vi "test_GetItemInfosFromProjectFile_SplitProjectTargetsSolution.vi"() -> (3 "Pass?":bool)   [LabVIEW 2019, in "Tests.SolutionBuilder.lvlib"]
uses:
  Tests.SolutionBuilder.lvlib
  SolutionBuilder/SolutionBuilder.lvclass
  SolutionBuilder/ProjectItem/ProjectItem.lvclass
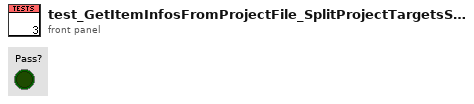
[diagram p1: front panel]
types:
  T1 = typedef "SolutionBuilder.lvlib/SolutionBuilder.lvclass/ProjectItemMap.ctl" = map{path, refnum<class "ProjectItem.lvclass">[]}
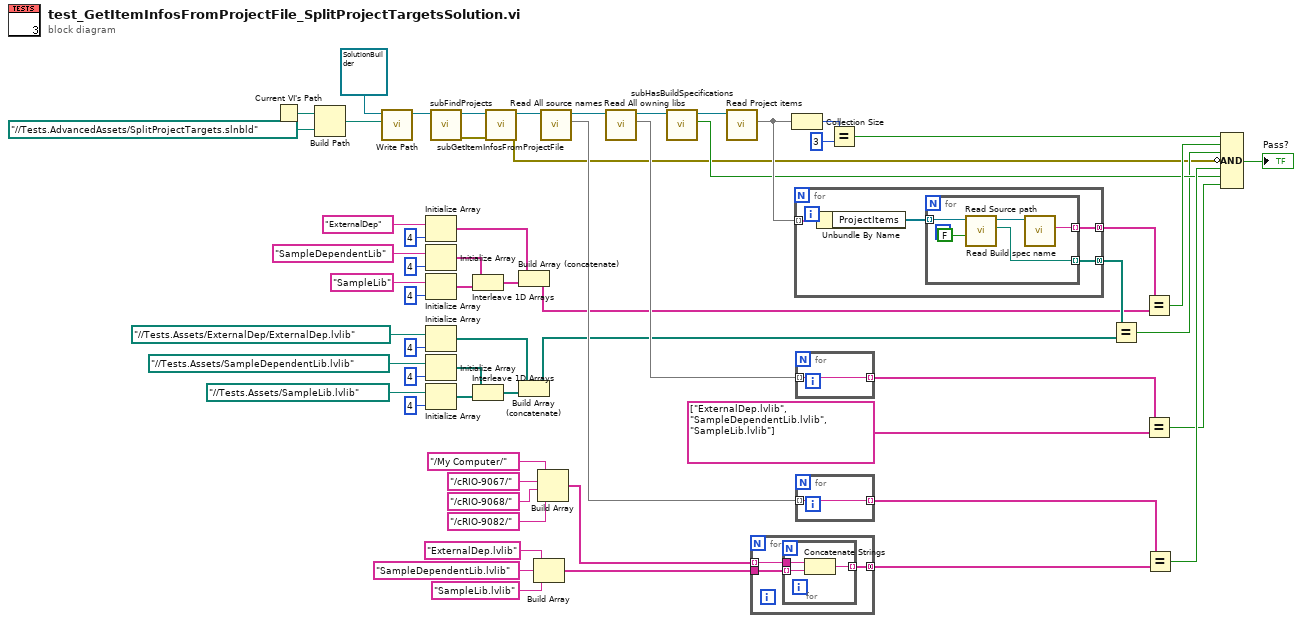
[diagram p0: block diagram]
diagram:
  n1 = Current VI's Path() -> (path=w58:path)
  n2 = Build Path(base path=w58, name or relative path=path "../../Tests.AdvancedAssets/SplitProjectTargets.slnbld" ("Path")) -> (appended path=w56:path)
  n3 = call "Write Path.vi"("Path"=w56, "SolutionBuilder in"=refnum<class "SolutionBuilder.lvclass"> refnum) -> ("SolutionBuilder out"=w60:refnum<class "SolutionBuilder.lvclass">)  [unwired: 9 in]
  n4 = Initialize Array("ExternalDep" ("Build spec name"), 4 ("dimension size")) -> (w24:string[])
  n5 = Initialize Array("SampleDependentLib" ("Build spec name"), 4 ("dimension size")) -> (w27:string[])
  n6 = Initialize Array("SampleLib" ("Build spec name"), 4 ("dimension size")) -> (w26:string[])
  n7 = Initialize Array(path "../../Tests.Assets/ExternalDep/ExternalDep.lvlib" ("Source path"), 4 ("dimension size")) -> (w22:path[])
  n8 = Initialize Array(path "../../Tests.Assets/SampleDependentLib.lvlib" ("Source path"), 4 ("dimension size")) -> (w19:path[])
  n9 = Initialize Array(path "../../Tests.Assets/SampleLib.lvlib" ("Source path"), 4 ("dimension size")) -> (w20:path[])
  n10 = call "subFindProjects.vi"("SolutionBuilder in"=w60) -> ("error out"=w35:errorcluster, "SolutionBuilder out"=w59:refnum<class "SolutionBuilder.lvclass">)  [unwired: 9 in]
  n11 = Interleave 1D Arrays(w27, w26) -> (w25:string[])
  n12 = Interleave 1D Arrays(w19, w20) -> (w21:path[])
  n13 = call "subGetItemInfosFromProjectFile.vi"("error in (no error)"=w35, "SolutionBuilder in"=w59) -> ("error out"=w34:errorcluster, "SolutionBuilder out"=w53:refnum<class "SolutionBuilder.lvclass">)  [unwired: 8 in]
  n14 = Build Array (concatenate)(w24, w25) -> (w23:string[])
  n15 = Build Array (concatenate)(w22, w21) -> (w12:path[])
  n16 = Build Array("ExternalDep.lvlib" ("Build spec name"), "SampleDependentLib.lvlib" ("Build spec name"), "SampleLib.lvlib" ("Build spec name")) -> (w3:string[])
  n17 = Build Array("/My Computer/" ("Build spec name"), "/cRIO-9067/" ("Build spec name"), "/cRIO-9068/" ("Build spec name"), "/cRIO-9082/" ("Build spec name")) -> (w4:string[])
  n18 = call "Read All source names.vi"("SolutionBuilder in"=w53) -> ("All source names"=w49:set{string}, "SolutionBuilder out"=w41:refnum<class "SolutionBuilder.lvclass">)  [unwired: 9 in]
  n19 = call "Read All owning libs.vi"("SolutionBuilder in"=w41) -> ("All owning libs"=w39:set{string}, "SolutionBuilder out"=w40:refnum<class "SolutionBuilder.lvclass">)  [unwired: 9 in]
  n20 = call "subHasBuildSpecifications.vi"("SolutionBuilder in"=w40) -> ("Has specs?"=w46:bool, "SolutionBuilder out"=w47:refnum<class "SolutionBuilder.lvclass">)  [unwired: 8 in, 1 out]
  n21 = call "Read Project items.vi"("SolutionBuilder in"=w47) -> ("Project items"=w52:T1)  [unwired: 9 in, 1 out]
  n22 = for {
    tunnel: w4 -> [w64] mode=indexing
    tunnel: w3 -> [w63]
    tunnel: [w62] -> w2 mode=concatenating
    n23 = for {
      tunnel: w64 -> [w67]
      tunnel: w63 -> [w66] mode=indexing
      tunnel: [w65] -> w62 mode=indexing
      n24 = Concatenate Strings(w67, w66) -> (w65:string)
    }
  }
  n25 = Collection Size(1:w52) -> (0:w55:i32)
  n26 = for {
    tunnel: w52 -> [w71] mode=indexing
    tunnel: [w70] -> w45 mode=concatenating
    tunnel: [w68] -> w43 mode=concatenating
    n27 = Unbundle By Name(w71) -> ("ProjectItems"=w69:refnum<class "ProjectItem.lvclass">[])
    n28 = for {
      tunnel: w69 -> [w74] mode=indexing
      tunnel: [w76] -> w70 mode=indexing
      tunnel: [w73] -> w68 mode=indexing
      n29 = call "Read Source path.vi"("Force abs path? (T)"=FALSE, "ProjectItem in"=w74) -> ("Source path"=w73:path, "ProjectItem out"=w75:refnum<class "ProjectItem.lvclass">)  [unwired: 8 in]
      n30 = call "Read Build spec name.vi"("ProjectItem in"=w75) -> ("Build spec name"=w76:string)  [unwired: 9 in, 1 out]
    }
  }
  n31 = for {
    tunnel: w39 -> [w77] mode=indexing
    tunnel: [w77] -> w38 mode=indexing
  }
  n32 = for {
    tunnel: w49 -> [w78] mode=indexing
    tunnel: [w78] -> w44 mode=indexing
  }
  n33 = Equal?(x=w55, y=3) -> (x = y?=w51:bool)
  n34 = Equal?(x=w43, y=w12) -> (x = y?=w42:bool)
  n35 = Equal?(x=w45, y=w23) -> (x = y?=w50:bool)
  n36 = Equal?(x=w38, y=string[] ["ExternalDep.lvlib", "SampleDependentLib.lvlib", "SampleLib.lvlib"] ("Array")) -> (x = y?=w36:bool)
  n37 = Equal?(x=w44, y=w2) -> (x = y?=w48:bool)
  n38 = Compound Arithmetic op=AND(w51, w50, w42, invert w34, w48, w46, w36) -> (→"Pass?":bool)
